vi "624FastTalonReadEncoderData.vi"(10 "Reset?":bool, 11 "CAN Talon SRX Ref":T1={"DeviceStatus"={"status"=FALSE, "code"=0, "source"=""}, "Type"=enum."PWM", "PWM"={"PWM Channel"=enum."PWM 1", "DeadBand"={"Name"="", "maxPositivePwm"=0, "minPositivePwm"=0, "centerPwm"=0, "maxNegativePwm"=0, "minNegativePwm"=0, "angularRange"=0}}, "CAN"={"Device Number"=0, "Control Mode"=enum."Percent VBus", "Semaphore"=refnum, "Max Vout"=12.0, "TalonSRX Control Mode"=enum."Percent VBus"}, "Invert"=FALSE}) -> (0 "Encoder Index Pin State":bool, 1 "Encoder Index Count":dbl, 2 "Encoder Velocity":dbl, 3 "Encoder Position":dbl, 4 "Encoder B Pin State":bool, 6 "Encoder A Pin State":bool)   [LabVIEW 2015]
uses:
  <vilib>/Rock Robotics/WPI/MotorControl/WPI_MotorControlDeviceRef.ctl
  <vilib>/Rock Robotics/WPI/MotorControl/WPI_MotorControlType.ctl
  <vilib>/Rock Robotics/SystemInterfaces/DIO/FPGA_DIOPWMChannel.ctl
  <vilib>/Rock Robotics/WPI/PWM/WPI_PWMDeadband.ctl
  <vilib>/Rock Robotics/WPI/CAN/Jaguar/SubVIs/WPI_CANJaguar_ControlMode.ctl
  <vilib>/Rock Robotics/WPI/CAN/TalonSRX/WPI_CANTalonSRX_APIControlMode.ctl
  <vilib>/Rock Robotics/WPI/CAN/TalonSRX/WPI_CANTalonSRX_MessageIDs.ctl
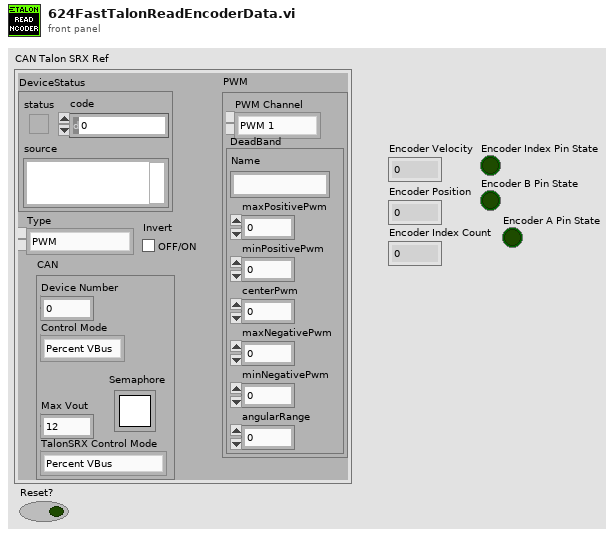
[diagram p1: front panel]
types:
  T1 = typedef "WPI_MotorControlDeviceRef.ctl" = cluster{"DeviceStatus":errorcluster, "Type":T2, "PWM":cluster{"PWM Channel":T3, "DeadBand":T4}, "CAN":cluster{"Device Number":u8, "Control Mode":T5, "Semaphore":T6, "Max Vout":dbl, "TalonSRX Control Mode":T7}, "Invert":bool}
  T2 = typedef "WPI_MotorControlType.ctl" = enum16{"PWM", "CAN", "CANTalonSRX"}
  T3 = typedef "FPGA_DIOPWMChannel.ctl" = enum8{"PWM 0", "PWM 1", "PWM 2", "PWM 3", "PWM 4", "PWM 5", "PWM 6", "PWM 7", "PWM 8", "PWM 9", "PWM MXP 0", "PWM MXP 1", "PWM MXP 2", "PWM MXP 3", "PWM MXP 4", "PWM MXP 5", "PWM MXP 6", "PWM MXP 7", "PWM MXP 8", "PWM MXP 9", "Invalid"}
  T4 = typedef "WPI_PWMDeadband.ctl" = cluster{"Name":string, "maxPositivePwm":i32, "minPositivePwm":i32, "centerPwm":i32, "maxNegativePwm":i32, "minNegativePwm":i32, "angularRange":u16}
  T5 = typedef "WPI_CANJaguar_ControlMode.ctl" = enum8{"Percent VBus", "Current", "Speed", "Position", "Voltage"}
  T6 = typedef "Semaphore RefNum" = refnum<k1>
  T7 = typedef "WPI_CANTalonSRX_APIControlMode.ctl" = enum8{"Percent VBus", "Speed", "Position", "Slave", "Unchanged / Invalid", "Voltage Compensation", "Current", "Motion Profile"}
  T8 = typedef "WPI_CANTalonSRX_MessageIDs.ctl" = u32
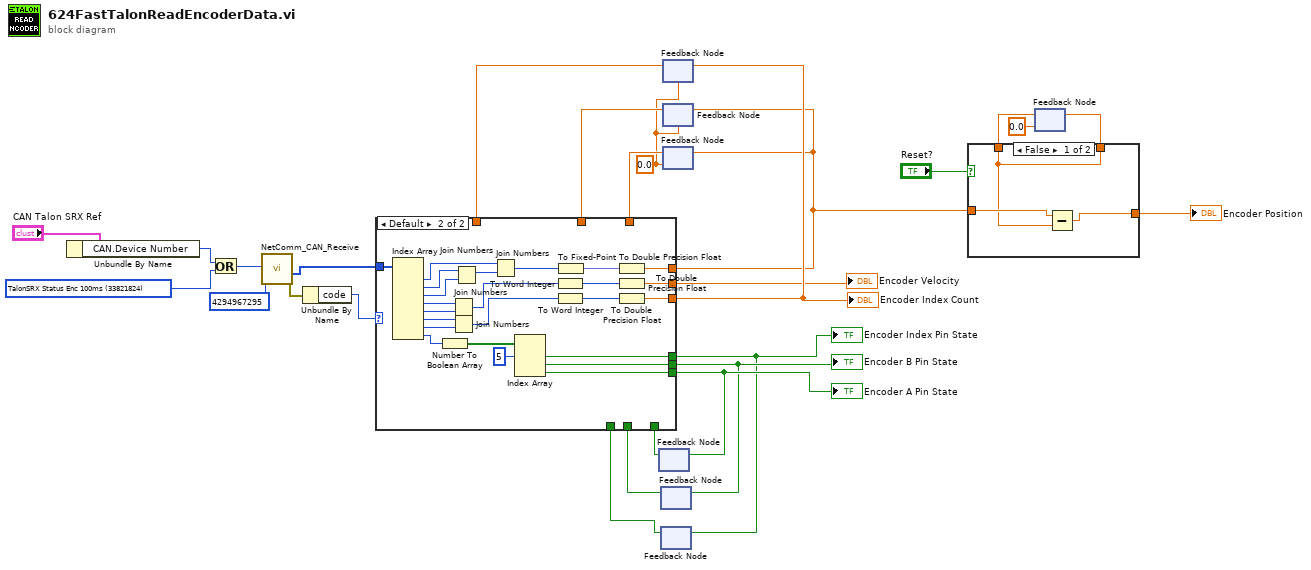
[diagram p0: block diagram]
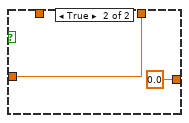
[diagram p2: hidden frame]
diagram:
  w1 = 0.0
  w23 = T8 33821824 items=["TalonSRX Control General 10ms"=33816576, "TalonSRX Control Rates Slow"=33816640, "TalonSRX Control ClearFlags Slow"=33816704, "TalonSRX Status General 10ms"=33821696, "TalonSRX Status Feedback 20ms"=33821760, "TalonSRX Status Enc 100ms"=33821824, "TalonSRX Status AinTempVbat 100ms"=33821888, "TalonSRX Status Startup Once"=33821952, "TalonSRX Status Debug"=33822080, "TalonSRX Config SetGainsSlot0 A"=33823808, "TalonSRX Config SetGainsSlot0 B"=33823872, "TalonSRX Config SetGainsSlot1 A"=33823936, "TalonSRX Config SetGainsSlot1 B"=33824000, "TalonSRX Config SetSoftLimits"=33824064, "TalonSRX Config WebControl"=33824128, "TalonSRX Param Request"=33822720, "TalonSRX Param Response"=33822784, "TalonSRX Param Set"=33822848]
  n1 = Unbundle By Name("CAN Talon SRX Ref") -> ("CAN.Device Number"=w24:u8)
  n2 = Or(x=w24, y=w23) -> (x .or. y?=w22:T8)
  n3 = call <vilib>:"NetComm_CAN_Receive.vi"("Message ID Mask"=u32 4294967295, "Message ID"=w22) -> ("error out"=w21:errorcluster, "Data"=w25:u8[])  [unwired: 1 in, 7 out]
  n4 = Unbundle By Name(w21) -> ("code"=w20:i32)
  n5 = feedback #1() -> (w13:bool)  [unwired: 1 in]
  n6 = feedback #2() -> (w11:bool)  [unwired: 1 in]
  n7 = feedback #3() -> (w9:bool)  [unwired: 1 in]
  n8 = feedback #4(w1) -> (w15:dbl)
  n9 = feedback #5(w1) -> (w17:dbl)
  n10 = feedback #6(w1) -> (w18:dbl)
  n11 = case shown="Default" w20 {
    tunnel: [w27 w48] -> w10
    tunnel: [w28 w47] -> w12
    tunnel: [w29 w46] -> w14
    tunnel: w25 -> [_ w36]
    tunnel: [w32 w35] -> w6
    tunnel: [w31 w34] -> w8
    tunnel: [w30 w33] -> w16
    tunnel: w18 -> [w32 _]
    tunnel: w17 -> [w31 _]
    tunnel: w15 -> [w30 _]
    tunnel: w13 -> [w29 _]
    tunnel: w11 -> [w28 _]
    tunnel: w9 -> [w27 _]
    frame -44087 {
    }
    frame Default {
      n12 = Index Array(array=w36) -> (element #1=w53:u8, element #2=w55:u8, element #3=w52:u8, element #4=w51:u8, element #5=w50:u8, element #6=w44:u8, element #7=w43:u8, element #8=w45:u8)  [unwired: 8 in]
      n13 = Number To Boolean Array(number=w45) -> (Boolean array=w56:bool[])
      n14 = Join Numbers(hi=w51, lo=w50) -> ((hi.lo)=w49:u16)
      n15 = Join Numbers(hi=w44, lo=w43) -> ((hi.lo)=w40:u16)
      n16 = Join Numbers(hi=w55, lo=w52) -> ((hi.lo)=w54:u16)
      n17 = Join Numbers(hi=w53, lo=w54) -> ((hi.lo)=w38:u32)
      n18 = Index Array(array=w56, index #1=5 ("index")) -> (element #1=w48:bool, element #2=w47:bool, element #3=w46:bool)  [unwired: 2 in]
      n19 = To Word Integer(number=w49) -> (16bit integer=w41:i16)
      n20 = To Word Integer(number=w40) -> (16bit integer=w39:i16)
      n21 = To Fixed-Point(number=w38) -> (fixed-point=w37:fxp<+/-,24,24>)  [unwired: 1 in]
      n22 = To Double Precision Float(number=w37) -> (double precision float=w35:dbl)
      n23 = To Double Precision Float(number=w41) -> (double precision float=w34:dbl)
      n24 = To Double Precision Float(number=w39) -> (double precision float=w33:dbl)
    }
  }
  "Encoder Velocity" <- w8
  "Encoder Index Count" <- w16
  "Encoder Index Pin State" <- w10
  "Encoder B Pin State" <- w12
  "Encoder A Pin State" <- w14
  n25 = feedback-in #1(w14) -> ()
  n26 = feedback-in #2(w12) -> ()
  n27 = feedback-in #3(w10) -> ()
  n28 = feedback-in #4(w16) -> ()
  n29 = feedback-in #5(w6) -> ()
  n30 = feedback-in #6(w6) -> ()
  n31 = feedback #7(0.0) -> (w4:dbl)
  n32 = case shown="False" "Reset?" {
    tunnel: w6 -> [w59 w61]
    tunnel: [w58 w61] -> w5
    tunnel: w4 -> [w58 _]
    tunnel: [w57 0.0] -> w3
    frame False {
      n33 = Subtract(x=w59, y=w58) -> (x-y=w57:dbl)
    }
    frame True {
    }
  }
  "Encoder Position" <- w3
  n34 = feedback-in #7(w5) -> ()
